vi "Stop and close.vi"(8 "error in (no error)":errorcluster, 11 "Scientifica XYZ Gen1 in":refnum<class "Scientifica XYZ Gen1.lvclass">) -> (0 "error out":errorcluster, 3 "Scientifica XYZ Gen1 out":refnum<class "Scientifica XYZ Gen1.lvclass">)   [LabVIEW 2020, in "TranslationStageClassStructure.lvlib" / "Scientifica XYZ Gen1.lvclass"]
uses:
  Scientifica XYZ Gen1.lvclass
  Scientifica XYZ Gen1.lvclass/Scientifica XYZ Gen1.ctl
  Serial Comms/Serial Comms/Serial Comms.lvclass
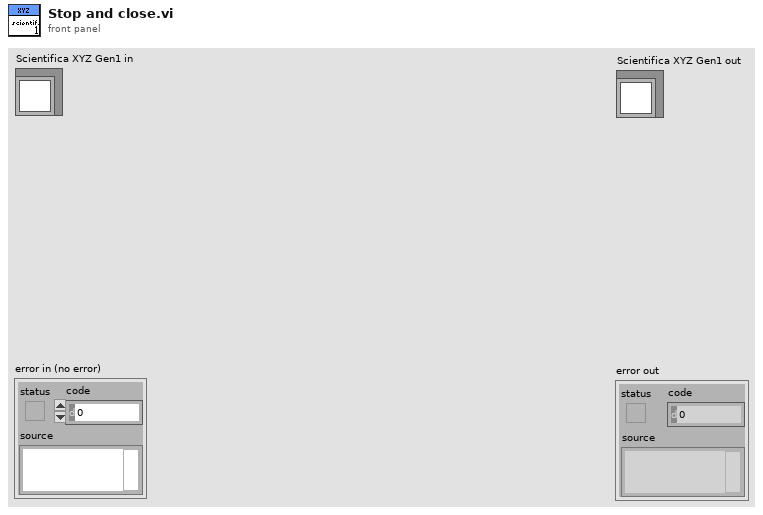
[diagram p1: front panel]
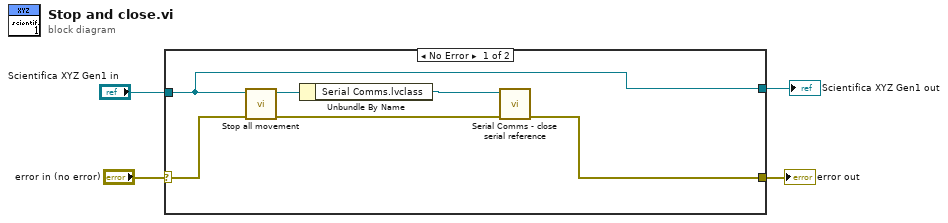
[diagram p0: block diagram]
diagram:
  n1 = case shown="No Error" "error in (no error)" {
    selector: "error in (no error)" -> [w10 w11]
    tunnel: [w6 w11] -> w3
    tunnel: "Scientifica XYZ Gen1 in" -> [w5 w12]
    tunnel: [w5 w12] -> w1
    frame No Error {
      n2 = call-dynamic "Stop all movement.vi"("error in (no error)"=w10, "Scientifica XYZ Gen1 in"=w5) -> ("error out"=w7:errorcluster, "Scientifica XYZ Gen1 out"=w9:refnum<class "Scientifica XYZ Gen1.lvclass">)  [unwired: 7 in, 1 out]
      n3 = Unbundle By Name(w9) -> ("Serial Comms.lvclass"=w8:refnum<class "Serial Comms.lvclass">)
      n4 = call "Serial Comms - close serial reference.vi"("error in (no error)"=w7, "Serial Comms in"=w8) -> ("error out"=w6:errorcluster)  [unwired: 8 in, 1 out]
    }
    frame Error {
    }
  }
  "error out" <- w3
  "Scientifica XYZ Gen1 out" <- w1
